vi "PDU Set All Outlets.vi"(8 "error in (no error)":errorcluster, 10 "State":bool[](array[boolean]), 11 "Orion PDU in":refnum<class "Orion PDU.lvclass">) -> (0 "error out":errorcluster, 2 "States out":bool[](array[boolean]), 3 "Orion PDU out":refnum<class "Orion PDU.lvclass">)   [LabVIEW 2022 SP3, in "Orion PDU.lvclass"]
uses:
  Orion PDU.lvclass
  C:/Development/rimas/RIMAS/Power Distribution/Power Distribution.lvclass
  Power Distribution.lvclass/Power Distribution.ctl
  Orion PDU.lvclass/Orion PDU.ctl
  Power Distribution.lvclass
panel:
  out "off command":string
  out "on command":string
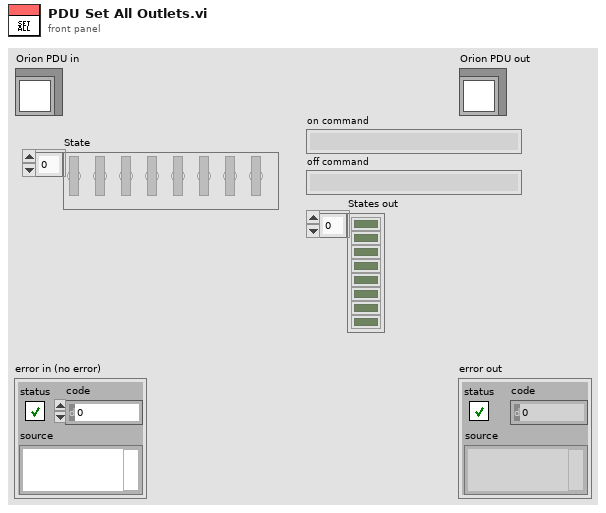
[diagram p1: front panel]
types:
  T1 = typedef "LabVIEWHTTPClient.lvlib/ClientHandle.ctl" = refnum<k1>
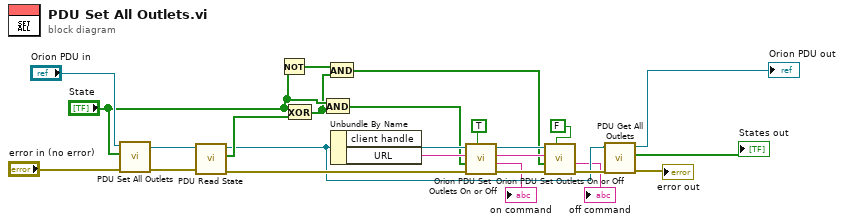
[diagram p0: block diagram]
diagram:
  n1 = call-parent "PDU Set All Outlets.vi"("error in (no error)"="error in (no error)", "State"="State", "Power Distribution in"="Orion PDU in") -> ("error out"=w23:errorcluster, "Power Distribution out"=w22:refnum<class "Orion PDU.lvclass">)  [unwired: 6 in, 1 out]
  n2 = call "PDU Read State.vi"("error in (no error)"=w23, "Power Distribution in"=w22) -> ("error out"=w16:errorcluster, "State"=w21:bool[], "Power Distribution out"=w8:refnum<class "Orion PDU.lvclass">)  [unwired: 7 in]
  n3 = Not(x="State") -> (.not. x?=w2:bool[])
  n4 = Exclusive Or(1:w21, 2:"State") -> (0:w3:bool[])
  n5 = And(x="State", y=w3) -> (x .and. y?=w17:bool[])
  n6 = And(x=w2, y=w3) -> (x .and. y?=w10:bool[])
  n7 = Unbundle By Name(w8) -> ("client handle"=w19:T1, "URL"=w18:string)
  n8 = call "Orion PDU Set Outlets On or Off.vi"("On?"=TRUE, "error in (no error)"=w16, "State"=w17, "addr"=w18, "client handle"=w19) -> ("error out"=w14:errorcluster, "command"=→"on command":string, "addr dup"=w12:string, "client handle out"=w13:T1)  [unwired: 3 in]
  n9 = call "Orion PDU Set Outlets On or Off.vi"("On?"=FALSE, "error in (no error)"=w14, "State"=w10, "addr"=w12, "client handle"=w13) -> ("error out"=w9:errorcluster, "command"=→"off command":string)  [unwired: 3 in, 2 out]
  n10 = call-dynamic "PDU Get All Outlets.vi"("error in (no error)"=w9, "Orion PDU in"=w8) -> ("error out"=→"error out":errorcluster, "States"=→"States out":bool[], "Orion PDU out"=→"Orion PDU out":refnum<class "Orion PDU.lvclass">)  [unwired: 7 in]
